vi "DAQmxTaskContainerPump_Start_Stop-Com-Exec.vi"(8 "error in (no error)":errorcluster, 9 "ControlQueue":refnum<queue>, 10 "data":variant, 11 "DAQmxTaksContainer_General in":refnum<class "DAQmxTaksContainer_General.lvclass">) -> (0 "error out":errorcluster, 3 "DAQmxTaksContainer_General out":refnum<class "DAQmxTaksContainer_General.lvclass">)   [LabVIEW 2018, in "DAQmxTaksContainer_General.lvclass"]
uses:
  DAQmxTaksContainer_General.lvclass
  dependecies/ControlsVIs/Clusters-def/SERVER-Commands.ctl
  dependecies/ControlsVIs/Clusters-def/ProtypeCommand-DAQmxReply.ctl
  DAQmxTask.lvclass
  Control/Control-Server/Control-Server.lvclass
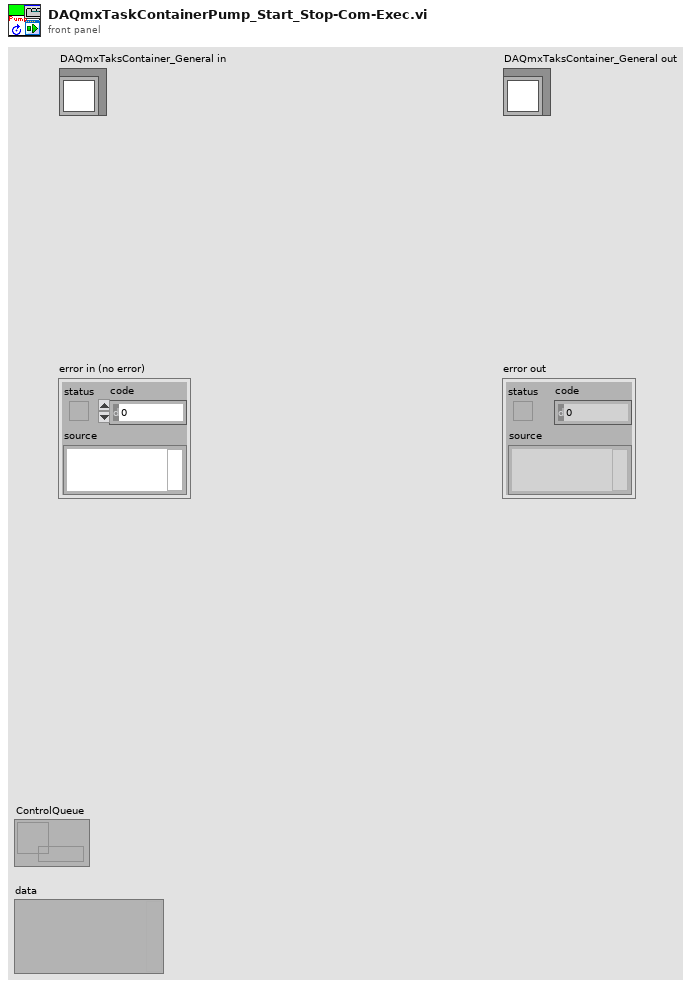
[diagram p1: front panel]
types:
  T1 = typedef "ProtypeCommand-DAQmxReply.ctl" = cluster{"On/Off":bool, "error out":errorcluster}
  T2 = typedef "Control-Server.lvclass/SERVER-Commands.ctl" = string
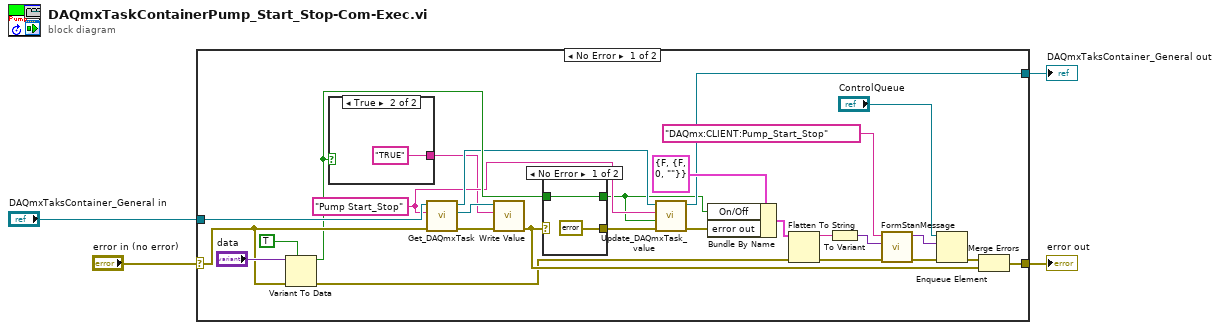
[diagram p0: block diagram]
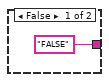
[diagram p2: hidden frame]
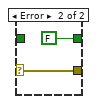
[diagram p3: hidden frame]
diagram:
  n1 = case shown="No Error" "error in (no error)" {
    selector: "error in (no error)" -> [w27 w39]
    tunnel: [w8 w38] -> w3
    tunnel: "DAQmxTaksContainer_General in" -> [w30 w38]
    tunnel: [w29 w39] -> w4
    frame No Error {
      w7 = "Pump Start_Stop" ("Task name")
      n2 = Variant To Data(error in=w27, type=TRUE, Variant="data") -> (data=w21:bool, error out=w18:errorcluster)
      n3 = case shown="True" w21 {
        tunnel: ["FALSE" ("Data") "TRUE" ("Data")] -> w5
        frame False {
        }
        frame True {
        }
      }
      n4 = call "Get_DAQmxTask.vi"("error in (no error)"=w27, "Task name"=w7, "DAQmxTaksContainer_General in"=w30) -> ("error out"=w26:errorcluster, "DAQmx Task"=w24:refnum<class "DAQmxTask.lvclass">, "DAQmxTaksContainer_General out"=w11:refnum<class "DAQmxTaksContainer_General.lvclass">)  [unwired: 6 in]
      n5 = call-dynamic "Write Value.vi"("error in (no error)"=w26, "Data"=w5, "DAQmxTask en entrée"=w24) -> ("error out"=w23:errorcluster)  [unwired: 7 in, 1 out]
      n6 = case shown="No Error" w23 {
        selector: w23 -> [_ w37]
        tunnel: [errorcluster {"status"=FALSE, "code"=5001, "source"="Relay key heater worked"} ("error constant") w37] -> w10
        tunnel: [w34 FALSE] -> w6
        tunnel: w21 -> [w34 _]
        frame No Error {
        }
        frame Error {
        }
      }
      n7 = call "Update_DAQmxTask_value.vi"("error in (no error)"=w10, "Value"=w6, "Task name"=w7, "DAQmxTaksContainer_General in"=w11) -> ("error out"=w9:errorcluster, "DAQmxTaksContainer_General out"=w8:refnum<class "DAQmxTaksContainer_General.lvclass">)  [unwired: 6 in]
      n8 = Bundle By Name(cluster=T1 {"On/Off"=FALSE, "error out"={"status"=FALSE, "code"=0, "source"=""}} ("output cluster"), "On/Off"=w6, "error out"=w9) -> (w19:T1)
      n9 = Flatten To String(anything=w19, error in (no error)=w18) -> (data string=w20:string, error out=w14:errorcluster)  [unwired: 2 in, 1 out]
      n10 = To Variant(anything=w20) -> (Variant=w15:variant)
      n11 = call "FormStanMessage.vi"("error in"=w14, "data"=w15, "Command"=T2 "DAQmx:CLIENT:Pump_Start_Stop" ("command")) -> ("error out"=w13:errorcluster, "message"=w12:variant)  [unwired: 7 in]
      n12 = Enqueue Element(queue="ControlQueue", element=w12, error in (no error)=w13) -> (error out=w17:errorcluster)  [unwired: 1 in, 2 out]
      n13 = Merge Errors(w17, w23) -> (w29:errorcluster)
    }
    frame Error {
    }
  }
  "error out" <- w4
  "DAQmxTaksContainer_General out" <- w3
